vi "FA Field Types.vi"(11 "Control Ref Array":refnum<vi>[](array[refnum])) -> (3 "Field Names Array":string[](array[string]))   [LabVIEW 2016, in "M1M3SupportEUI_Views.lvlib"]
uses:
  M1M3SupportEUI_Views.lvlib
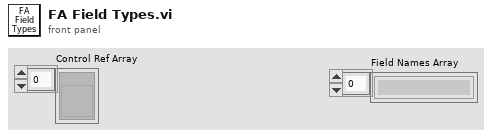
[diagram p1: front panel]
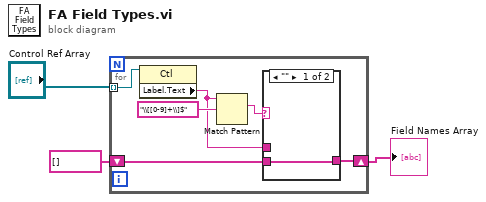
[diagram p0: block diagram]
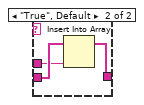
[diagram p2: hidden frame]
diagram:
  n1 = for {
    tunnel: "Control Ref Array" -> [w9] mode=indexing
    shift-right: [w4] -> w1
    shift-left: string[] [] -> [w6]
    n2 = property class="Ctl"(reference=w9) -> ("Label.Text"=w5:string)  [unwired: 1 in, 2 out]
    n3 = Match Pattern(string=w5, regular expression="\\[[0-9]+\\]$") -> (match substring=w7:string)  [unwired: 1 in, 3 out]
    n4 = case shown="\"\"" w7 {
      tunnel: w6 -> [w10 w13]
      tunnel: w5 -> [_ w12]
      tunnel: [w10 w11] -> w4
      frame "" {
      }
      frame "True", Default {
        n5 = Insert Into Array(array=w13, new element=w12) -> (w11:string[])  [unwired: 1 in]
      }
    }
  }
  "Field Names Array" <- w1
